vi "Extract Expt Parameters from YAML notes.vi"(8 "error in (no error)":errorcluster, 11 "YAML Comments IN":string="YAML Comments IN") -> (0 "error out":errorcluster, 1 "device details":string[][](array[string]), 2 "wiring":string[][](array[string]), 3 "Experiment Parameters From 1st ITX":T1)   [LabVIEW 2016]
uses:
  <userlib>/LevyLab/PLYM/YAML.lvclass
panel:
  out "lockin contents":string[][](array[string])
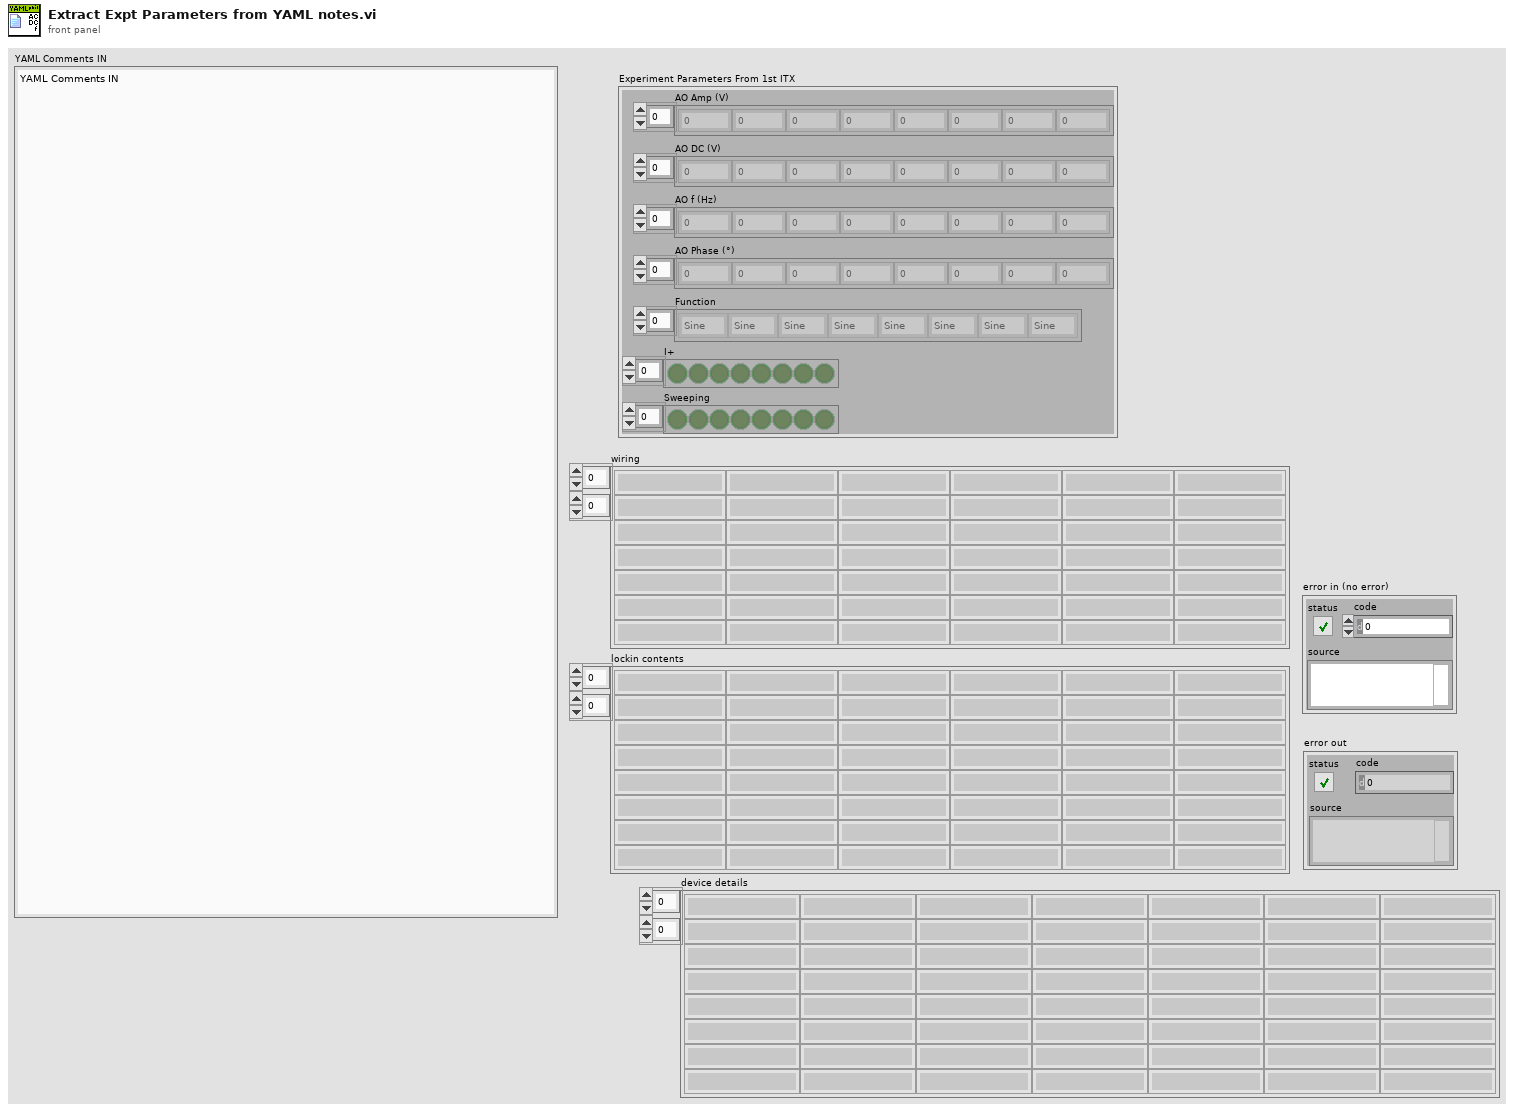
[diagram p1: front panel]
types:
  T1 = cluster{"AO Amp (V)":dbl[], "AO DC (V)":dbl[], "AO f (Hz)":dbl[], "AO Phase (°)":dbl[], "Function":enum16{"Sine", "Triangle", "Square", "Sawtooth"}[], "I+":bool[], "Sweeping":bool[]}
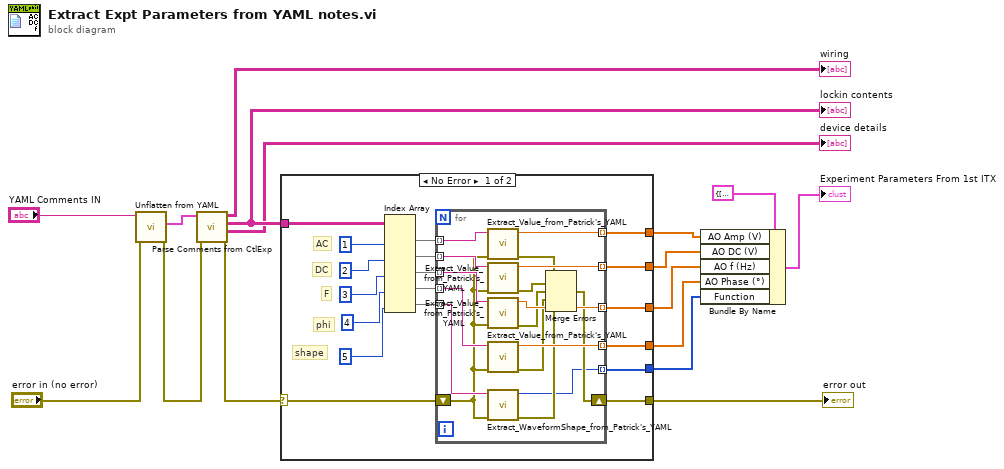
[diagram p0: block diagram]
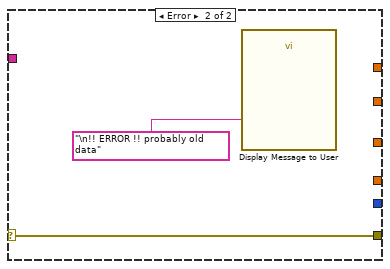
[diagram p2: hidden frame]
diagram:
  n1 = call <userlib>:"Unflatten from YAML.vi"("error in (no error)"="error in (no error)", "YAML String"="YAML Comments IN") -> ("error out"=w1:errorcluster, "YAML Dictionary Items"=w4:cluster{"key":variant, "value":variant}[])  [unwired: 7 in, 1 out]
  n2 = call <userlib>:"Parse Comments from CtlExp.vi"("error in"=w1, "dictionary from yaml parser"=w4) -> ("error out"=w12:errorcluster, "device details"=→"device details":string[][], "lockin contents"=w11:string[][], "wiring"=→"wiring":string[][])  [unwired: 5 in]
  "lockin contents" <- w11
  n3 = case shown="No Error" w12 {
    selector: w12 -> [w21 w52]
    tunnel: w11 -> [w34 _]
    tunnel: [w27 _] -> w15
    tunnel: [w26 _] -> w14
    tunnel: [w25 _] -> w13
    tunnel: [w20 w52] -> w9
    tunnel: [w22 _] -> w8
    tunnel: [w17 _] -> w7
    frame No Error {
      # "shape"
      # "phi"
      # "F"
      # "DC"
      # "AC"
      n4 = Index Array(array=w34, index (col) #1=1 ("disabled index (col)"), index (col) #2=2 ("index (col)"), index (col) #3=3 ("index (col)"), index (col) #4=4 ("index (col)"), index (col) #5=5 ("index (col)")) -> (element #1=w32:string[], element #2=w31:string[], element #3=w28:string[], element #4=w23:string[], element #5=w18:string[])  [unwired: 5 in]
      n5 = for {
        tunnel: w32 -> [w51] mode=indexing
        tunnel: w31 -> [w48] mode=indexing
        tunnel: [w49] -> w26 mode=indexing
        tunnel: [w50] -> w27 mode=indexing
        tunnel: w28 -> [w47] mode=indexing
        tunnel: [w46] -> w25 mode=indexing
        tunnel: w23 -> [w45] mode=indexing
        tunnel: [w44] -> w22 mode=indexing
        shift-right: [w39] -> w20
        shift-left: w21 -> [w37]
        tunnel: w18 -> [w38] mode=indexing
        tunnel: [w35] -> w17 mode=indexing
        n6 = call <userlib>:"Extract_Value_from_Patrick's_YAML.vi"("error in (no error)"=w37, "String"=w51) -> ("error out"=w43:errorcluster, "Numeric"=w50:dbl)  [unwired: 8 in]
        n7 = call <userlib>:"Extract_Value_from_Patrick's_YAML.vi"("error in (no error)"=w37, "String"=w48) -> ("error out"=w42:errorcluster, "Numeric"=w49:dbl)  [unwired: 8 in]
        n8 = call <userlib>:"Extract_Value_from_Patrick's_YAML.vi"("error in (no error)"=w37, "String"=w47) -> ("error out"=w41:errorcluster, "Numeric"=w46:dbl)  [unwired: 8 in]
        n9 = call <userlib>:"Extract_Value_from_Patrick's_YAML.vi"("error in (no error)"=w37, "String"=w45) -> ("error out"=w40:errorcluster, "Numeric"=w44:dbl)  [unwired: 8 in]
        n10 = call <userlib>:"Extract_WaveformShape_from_Patrick's_YAML.vi"("error in (no error)"=w37, "String"=w38) -> ("error out"=w36:errorcluster, "data"=w35:enum16{"Sine", "Triangle", "Square", "Sawtooth"})  [unwired: 8 in]
        n11 = Merge Errors(w43, w42, w41, w40, w36) -> (w39:errorcluster)
      }
    }
    frame Error {
      n12 = call "Display Message to User"("Message"="\n!! ERROR !! probably old data" ("string")) -> ()  [unwired: 9 in, 2 out]
    }
  }
  "error out" <- w9
  n13 = Bundle By Name(cluster=T1 {"AO Amp (V)"=[0.01, 0.0, 0.0, 0.0, 0.0, 0.0, 0.0, 0.0], "AO DC (V)"=[0.0, 0.0, 0.0, 0.0, 0.0, 0.0, 0.0, 0.0], "AO f (Hz)"=[13.1, 13.0, 13.0, 13.0, 13.0, 13.0, 13.0, 13.0], "AO Phase (°)"=[0.0, 0.0, 0.0, 0.0, 0.0, 0.0, 0.0, 0.0], "Function"=[enum."Sine", enum."Sine", enum."Sine", enum."Sine", enum."Sine", enum."Sine", enum."Sine", enum."Sine"], "I+"=[], "Sweeping"=[]} ("Channels: AO"), "AO Amp (V)"=w15, "AO DC (V)"=w14, "AO f (Hz)"=w13, "AO Phase (°)"=w8, "Function"=w7) -> (→"Experiment Parameters From 1st ITX":T1)
